vi "Read Double Direct.vi"(8 "error in (no error)":errorcluster, 9 "Timeout (ms)":i32, 11 "CIFTag in":refnum<class "CIF_CIPC_Chn_Double.lvclass">) -> (0 "error out":errorcluster, 1 "timed out?":bool, 2 "Data":dbl, 3 "CIFTag out":refnum<class "CIF_CIPC_Chn_Double.lvclass">)   [LabVIEW 2021, in "CIF_CIPC_Chn_Double.lvclass"]
uses:
  CIF_CIPC_Chn_Double.lvclass
  D:/dev/Packages/CIF_Channels_Core/src/CIFChannels/CIFChannels.lvclass
  D:/dev/Packages/CIF_Channels_Core/src/CIPC_Channels/CIF_CIPC_Chan/CIF_CIPC_Chn.lvclass
  CIFChannels/CIFChannels.lvclass/CIFChannels.ctl
  CIFChannels/Typedef/Channel State.ctl
  CIFChannels/Typedef/Direction.ctl
  CIF_CIPC_Chn_Double.lvclass/CIF_CIPC_Chn_Double.ctl
  CIF_CIPC_Chan/CIF_CIPC_Chn.lvclass/CIF_CIPC_Chn.ctl
  <vilib>/CIF Foundation/CIF CIPC/TypeDefs/Data Element Details.ctl
  ed3b2614-2534-48bf-9d55-8103b1731be4.vi
  9835d51f-0a03-4fca-8b65-57ff329e3dc0.vi
  48c6cd7f-44dd-4d44-b4f8-9fb6ce13bfd2.vi
  9d42b1fa-14d5-40ea-8bb3-5a2065a11a1e.vi
  9fddd408-4685-490b-9ae7-4ba7fd4a7e7d.vi
  dd9db9cb-e8a4-4889-9d38-6a9c25c23114.vi
  322a00c8-bb5b-4919-ac68-9d1b04b85b95.vi
  43cc0021-f1c2-48da-bdf0-2456dac13c8c.vi
  ff0ef007-ba63-4493-b728-c38daa37d23e.vi
  cc24c00a-8a47-44d0-84f9-fbc2e6207c11.vi
  de648ecb-ca24-4a8e-b28e-520279f4721e.vi
  CIF_CIPC_Chan/Accessors/Read Buffer Configuration.vi
  CIF_CIPC_Chan/Accessors/Read Data Type.vi
  CIFChannels/Accessors/Read Channel State.vi
  CIFChannels/Accessors/Read Direction.vi
  CIFChannels/Accessors/Read Tag Forced.vi
  CIFChannels/Accessors/Write Channel State.vi
  CIFChannels/Accessors/Read Tag Disconnect Behavior.vi
  <vilib>/CIF Foundation/CIF CIPC/SubVIs/Wait For N Elements Available.vi
  <vilib>/CIF Foundation/CIF CIPC/SubVIs/Get Element Read Position.vi
  <vilib>/CIF Foundation/CIF CIPC/SubVIs/Check Error.vi
  <vilib>/CIF Foundation/CIF CIPC/SubVIs/Get dll Path.vi
  <vilib>/CIF Foundation/CIF CIPC/SubVIs/Set Element Read Position.vi
  CIF_CIPC_Chan/CIF_CIPC_Chn.lvclass
  <vilib>/CIF Foundation/CIF CIPC/SubVIs/Check Error Core.vi
  CIFChannels/CIFChannels.lvclass
  <vilib>/CIF Foundation/CIF CIPC/CIF_NI_CIPC.lvlib
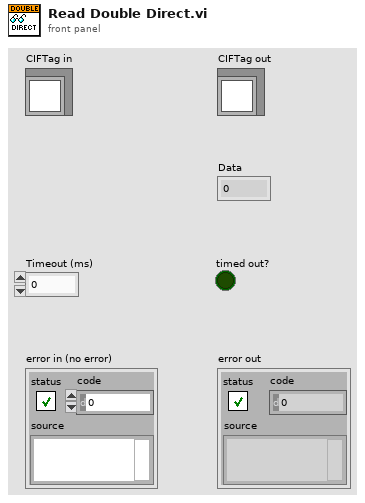
[diagram p1: front panel]
types:
  T1 = typedef "CIFChannels.lvclass/Channel State.ctl" = enum16{"Creating", "Disconnected", "Connecting", "Connected", "Destroyed"}
  T2 = typedef "CIFChannels.lvclass/Direction.ctl" = enum16{"Publisher", "Subscriber"}
  T3 = typedef "CIF_NI_CIPC.lvlib/Data Element Details.ctl" = cluster{"Bytes to Read":u32, "Element Offset":u32}
  T4 = typedef "CIF_CIPC_Chn.lvclass/Buffer Configuration Data.ctl" = cluster{"Total Size":u32, "Read Size":u32, "Read Offset":u32, "CIPC BP References":T5, "CIPC Backpressure Names":T6, "Override CIPC Name":string, "Encoder Data":string}
  T5 = typedef "CIF_NI_CIPC.lvlib/Backpressure References.ctl" = cluster{"CIPC Reference":u64, "CIPC BP Reference":u64}
  T6 = typedef "CIF_NI_CIPC.lvlib/Backpressure Names.ctl" = cluster{"CIPC Name":string, "CIPC BP Name":string}
  T7 = typedef "NI_Data Type.lvlib/Data Type.ctl" = enum8{"Invalid Type", "Void", "I8", "I16", "I32", "I64", "U8", "U16", "U32", "U64", "Single Float", "Double Float", "Extended Float", "Single Complex", "Double Complex", "Extended Complex", "Enum U8", "Enum U16", "Enum U32", "Enum U64", "Single Float With Unit", "Double Float With Unit", "Extended Float With Unit", "Single Complex with Unit", "Double Complex with Unit", "Extended Complex with Unit", "Boolean", "String", "Path", "Picture", "Tag", "Array", "Cluster", "Variant", "LV Variant", "Waveform", "Timestamp", "Digital Waveform", "Digital Data", "ExpressData", "Refnum", "External Data", "VI", "Poly VI", "LabVIEW Class Instance", "Fixed Point", "Set Collection", "Map Collection"}
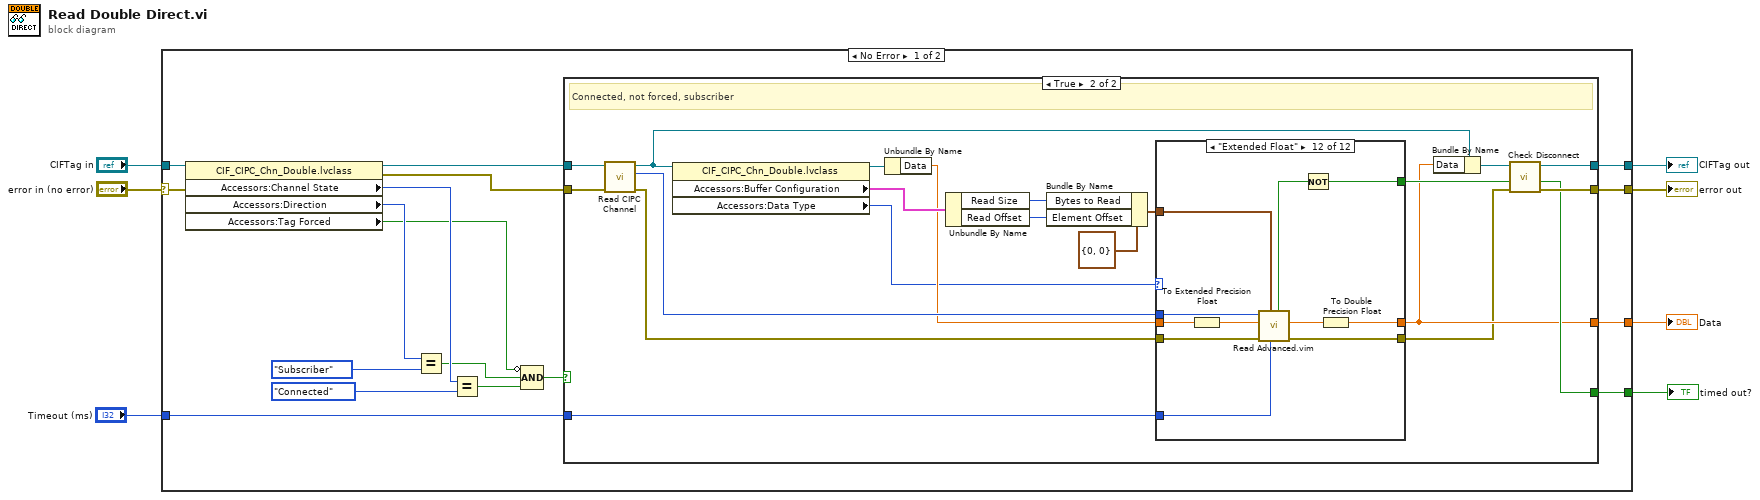
[diagram p0: block diagram]
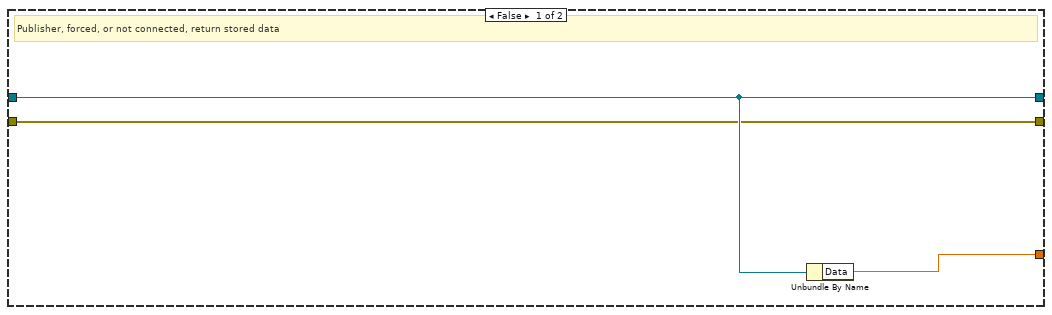
[diagram p2: hidden frame]
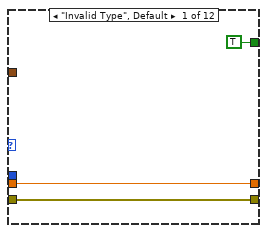
[diagram p3: hidden frame]
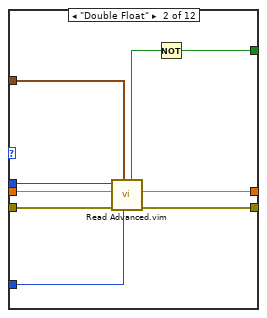
[diagram p4: hidden frame]
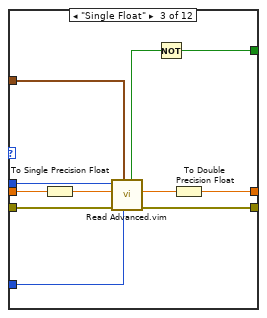
[diagram p5: hidden frame]
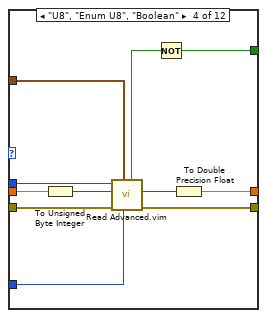
[diagram p6: hidden frame]
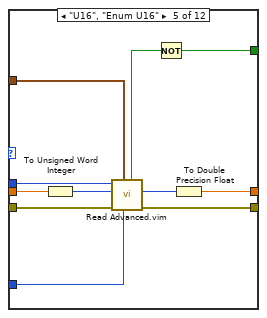
[diagram p7: hidden frame]
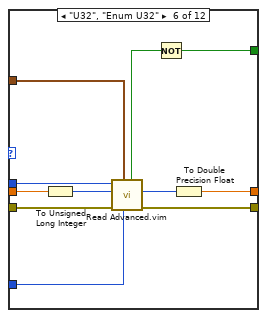
[diagram p8: hidden frame]
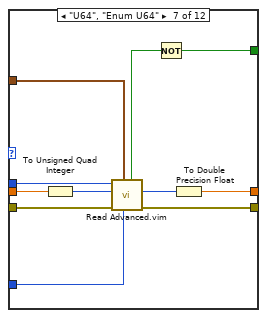
[diagram p9: hidden frame]
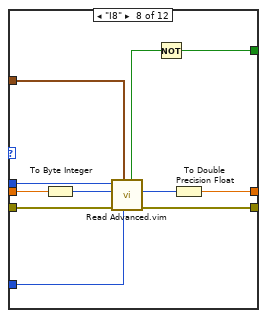
[diagram p10: hidden frame]
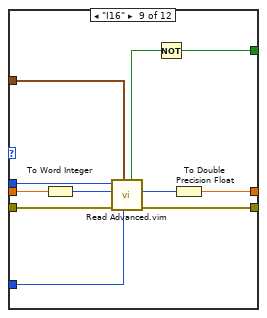
[diagram p11: hidden frame]
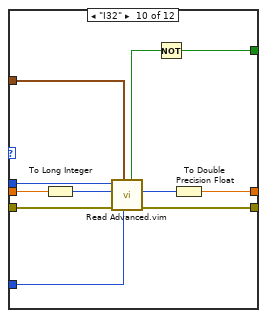
[diagram p12: hidden frame]
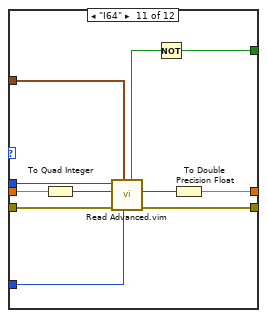
[diagram p13: hidden frame]
diagram:
  n1 = case shown="No Error" "error in (no error)" {
    selector: "error in (no error)" -> [w21 w172]
    tunnel: [w10 w172] -> w6
    tunnel: [w11 w171] -> w4
    tunnel: "CIFTag in" -> [w22 w171]
    tunnel: [w24 _] -> w3
    tunnel: [w23 _] -> w2
    tunnel: "Timeout (ms)" -> [w9 _]
    frame No Error {
      n2 = property class="CIF_CIPC_Chn_Double.lvclass"(reference=w22, error in=w21) -> (reference out=w20:refnum<class "CIF_CIPC_Chn_Double.lvclass">, error out=w19:errorcluster, "Accessors:Channel State"=w16:T1, "Accessors:Direction"=w18:T2, "Accessors:Tag Forced"=w8:bool)
      n3 = Equal?(x=w18, y=Direction."Subscriber") -> (x = y?=w12:bool)
      n4 = Equal?(x=w16, y=Channel_State."Connected") -> (x = y?=w14:bool)
      n5 = Compound Arithmetic op=AND(invert w8, w12, w14) -> (w13:bool)
      n6 = case shown="True" w13 {
        tunnel: [_ w42] -> w24
        tunnel: [w27 w31] -> w23
        tunnel: w19 -> [w25 w47]
        tunnel: w20 -> [w26 w48]
        tunnel: [w26 w45] -> w11
        tunnel: [w25 w46] -> w10
        tunnel: w9 -> [_ w32]
        frame False {
          # "Publisher, forced, or not connected, return stored data"
          n7 = Unbundle By Name(w26) -> ("Data"=w27:dbl)
        }
        frame True {
          # "Connected, not forced, subscriber"
          n8 = call "Read CIPC Channel.vi"("error in (no error)"=w47, "CIFTag in"=w48) -> ("error out"=w33:errorcluster, "CIPC Channel"=w34:u64, "CIFTag out"=w41:refnum<class "CIF_CIPC_Chn_Double.lvclass">)  [unwired: 7 in]
          n9 = property class="CIF_CIPC_Chn_Double.lvclass"(reference=w41) -> (reference out=w40:refnum<class "CIF_CIPC_Chn_Double.lvclass">, "Accessors:Buffer Configuration"=w36:T4, "Accessors:Data Type"=w28:T7)  [unwired: 1 in, 1 out]
          n10 = Unbundle By Name(w40) -> ("Data"=w30:dbl)
          n11 = Unbundle By Name(w36) -> ("Read Size"=w38:u32, "Read Offset"=w37:u32)
          n12 = Bundle By Name(cluster=T3 {"Bytes to Read"=0, "Element Offset"=0} ("Data Element"), "Bytes to Read"=w38, "Element Offset"=w37) -> (w35:T3)
          n13 = case shown="\"Extended Float\"" w28 {
            tunnel: [TRUE w60 w71 w82 w93 w104 w115 w126 w137 w148 w159 w170] -> w43
            tunnel: w35 -> [_ w59 w70 w81 w92 w103 w114 w125 w136 w147 w158 w169]
            tunnel: w34 -> [_ w58 w69 w80 w91 w102 w113 w124 w135 w146 w157 w168]
            tunnel: w33 -> [w50 w57 w68 w79 w90 w101 w112 w123 w134 w145 w156 w167]
            tunnel: w32 -> [_ w56 w67 w78 w89 w100 w111 w122 w133 w144 w155 w166]
            tunnel: [w51 w54 w61 w72 w83 w94 w105 w116 w127 w138 w149 w160] -> w31
            tunnel: w30 -> [w51 w53 w64 w75 w86 w97 w108 w119 w130 w141 w152 w163]
            tunnel: [w50 w52 w63 w74 w85 w96 w107 w118 w129 w140 w151 w162] -> w29
            frame "Invalid Type", Default {
            }
            frame "Double Float" {
              n14 = call "Read Advanced.vim"("Timeout (ns)"=w56, "Data Element"=w59, "error in (no error)"=w57, "Data in"=w53, "CIPC Reference in"=w58) -> ("error out"=w52:errorcluster, "Data out"=w54:dbl, "Success"=w55:bool)  [unwired: 2 in, 2 out]
              n15 = Not(x=w55) -> (.not. x?=w60:bool)
            }
            frame "Single Float" {
              n16 = To Single Precision Float(number=w64) -> (single precision float=w62:sgl)
              n17 = call "Read Advanced.vim"("Timeout (ns)"=w67, "Data Element"=w70, "error in (no error)"=w68, "Data in"=w62, "CIPC Reference in"=w69) -> ("error out"=w63:errorcluster, "Data out"=w65:sgl, "Success"=w66:bool)  [unwired: 2 in, 2 out]
              n18 = Not(x=w66) -> (.not. x?=w71:bool)
              n19 = To Double Precision Float(number=w65) -> (double precision float=w61:dbl)
            }
            frame "U8", "Enum U8", "Boolean" {
              n20 = To Unsigned Byte Integer(number=w75) -> (unsigned 8bit integer=w73:u8)
              n21 = call "Read Advanced.vim"("Timeout (ns)"=w78, "Data Element"=w81, "error in (no error)"=w79, "Data in"=w73, "CIPC Reference in"=w80) -> ("error out"=w74:errorcluster, "Data out"=w76:u8, "Success"=w77:bool)  [unwired: 2 in, 2 out]
              n22 = Not(x=w77) -> (.not. x?=w82:bool)
              n23 = To Double Precision Float(number=w76) -> (double precision float=w72:dbl)
            }
            frame "U16", "Enum U16" {
              n24 = To Unsigned Word Integer(number=w86) -> (unsigned 16bit integer=w84:u16)
              n25 = call "Read Advanced.vim"("Timeout (ns)"=w89, "Data Element"=w92, "error in (no error)"=w90, "Data in"=w84, "CIPC Reference in"=w91) -> ("error out"=w85:errorcluster, "Data out"=w87:u16, "Success"=w88:bool)  [unwired: 2 in, 2 out]
              n26 = Not(x=w88) -> (.not. x?=w93:bool)
              n27 = To Double Precision Float(number=w87) -> (double precision float=w83:dbl)
            }
            frame "U32", "Enum U32" {
              n28 = To Unsigned Long Integer(number=w97) -> (unsigned 32bit integer=w95:u32)
              n29 = call "Read Advanced.vim"("Timeout (ns)"=w100, "Data Element"=w103, "error in (no error)"=w101, "Data in"=w95, "CIPC Reference in"=w102) -> ("error out"=w96:errorcluster, "Data out"=w98:u32, "Success"=w99:bool)  [unwired: 2 in, 2 out]
              n30 = Not(x=w99) -> (.not. x?=w104:bool)
              n31 = To Double Precision Float(number=w98) -> (double precision float=w94:dbl)
            }
            frame "U64", "Enum U64" {
              n32 = To Unsigned Quad Integer(1:w108) -> (0:w106:u64)
              n33 = call "Read Advanced.vim"("Timeout (ns)"=w111, "Data Element"=w114, "error in (no error)"=w112, "Data in"=w106, "CIPC Reference in"=w113) -> ("error out"=w107:errorcluster, "Data out"=w109:u64, "Success"=w110:bool)  [unwired: 2 in, 2 out]
              n34 = Not(x=w110) -> (.not. x?=w115:bool)
              n35 = To Double Precision Float(number=w109) -> (double precision float=w105:dbl)
            }
            frame "I8" {
              n36 = To Byte Integer(number=w119) -> (8bit integer=w117:i8)
              n37 = call "Read Advanced.vim"("Timeout (ns)"=w122, "Data Element"=w125, "error in (no error)"=w123, "Data in"=w117, "CIPC Reference in"=w124) -> ("error out"=w118:errorcluster, "Data out"=w120:i8, "Success"=w121:bool)  [unwired: 2 in, 2 out]
              n38 = Not(x=w121) -> (.not. x?=w126:bool)
              n39 = To Double Precision Float(number=w120) -> (double precision float=w116:dbl)
            }
            frame "I16" {
              n40 = To Word Integer(number=w130) -> (16bit integer=w128:i16)
              n41 = call "Read Advanced.vim"("Timeout (ns)"=w133, "Data Element"=w136, "error in (no error)"=w134, "Data in"=w128, "CIPC Reference in"=w135) -> ("error out"=w129:errorcluster, "Data out"=w131:i16, "Success"=w132:bool)  [unwired: 2 in, 2 out]
              n42 = Not(x=w132) -> (.not. x?=w137:bool)
              n43 = To Double Precision Float(number=w131) -> (double precision float=w127:dbl)
            }
            frame "I32" {
              n44 = To Long Integer(number=w141) -> (32bit integer=w139:i32)
              n45 = call "Read Advanced.vim"("Timeout (ns)"=w144, "Data Element"=w147, "error in (no error)"=w145, "Data in"=w139, "CIPC Reference in"=w146) -> ("error out"=w140:errorcluster, "Data out"=w142:i32, "Success"=w143:bool)  [unwired: 2 in, 2 out]
              n46 = Not(x=w143) -> (.not. x?=w148:bool)
              n47 = To Double Precision Float(number=w142) -> (double precision float=w138:dbl)
            }
            frame "I64" {
              n48 = To Quad Integer(1:w152) -> (0:w150:i64)
              n49 = call "Read Advanced.vim"("Timeout (ns)"=w155, "Data Element"=w158, "error in (no error)"=w156, "Data in"=w150, "CIPC Reference in"=w157) -> ("error out"=w151:errorcluster, "Data out"=w153:i64, "Success"=w154:bool)  [unwired: 2 in, 2 out]
              n50 = Not(x=w154) -> (.not. x?=w159:bool)
              n51 = To Double Precision Float(number=w153) -> (double precision float=w149:dbl)
            }
            frame "Extended Float" {
              n52 = To Extended Precision Float(1:w163) -> (0:w161:ext)
              n53 = call "Read Advanced.vim"("Timeout (ns)"=w166, "Data Element"=w169, "error in (no error)"=w167, "Data in"=w161, "CIPC Reference in"=w168) -> ("error out"=w162:errorcluster, "Data out"=w164:ext, "Success"=w165:bool)  [unwired: 2 in, 2 out]
              n54 = Not(x=w165) -> (.not. x?=w170:bool)
              n55 = To Double Precision Float(number=w164) -> (double precision float=w160:dbl)
            }
          }
          n56 = Bundle By Name(cluster=w41, "Data"=w31) -> (w44:refnum<class "CIF_CIPC_Chn_Double.lvclass">)
          n57 = call "Check Disconnect.vi"("error in (no error)"=w29, "timeout in"=w43, "CIFTag in"=w44) -> ("error out"=w46:errorcluster, "timeout out"=w42:bool, "CIFTag out"=w45:refnum<class "CIF_CIPC_Chn_Double.lvclass">)  [unwired: 5 in, 1 out]
        }
      }
    }
    frame Error {
    }
  }
  "error out" <- w6
  "CIFTag out" <- w4
  "timed out?" <- w3
  "Data" <- w2
